vi "New_FPGA_Hex_Gen.vi"(9 "Laser(V)":dbl[](array[numeric]), 11 "Chirp Parameters":T21) -> (0 "distortion_corr":dbl, 1 "timings_offsets":dbl[](array[numeric]), 2 "HEX Array":string[](array[string]), 3 "Interrupted":bool)   [LabVIEW 2020]
uses:
  Controls/Frequency Record.ctl
  Global Variables/General Globals.vi
  Typedefs/HW config states enum.ctl
  Controls/Pockels_Galvo_Params.ctl
  Typedefs/Chirp_ABCD.ctl
  Typedefs/Cam VidRec HW config setup cluster.ctl
  Typedefs/Control Sys HW config cluster.ctl
  <vilib>/userDefined/High Color/nirio_resource_hc.ctl
  Typedefs/FPGA input type AC-DC.ctl
  Typedefs/DAQmx physical channels cluster.ctl
  Typedefs/Encoder config cluster.ctl
  Typedefs/Laser 1 config cluster.ctl
  Typedefs/PreChirper 1 config cluster.ctl
  Typedefs/Laser Power Control HW config.ctl
  Typedefs/Triggers HW config.ctl
  Typedefs/Hardware Configuration settings.ctl
  RIG-SPECIFIC FILES/FPGA Refs/FPGA Ref.ctl
  Typedefs/DAQ FPGA system config.ctl
  Typedefs/CTRL system config.ctl
  Typedefs/System Configuration.ctl
  Typedefs/DAQ FPGA HW config cluster.ctl
  Typedefs/PMT Control Voltage limits.ctl
  Peripherals Control/XYZ Stage/Control/typedefs/XYZControlConfig.ctl
  Typedefs/Comms Type.ctl
  Typedefs/Peripherals comms config cluster.ctl
panel:
  in  "System Config":T1={"Laser wavelength (nm)"=920.0, "DAQ FPGA System"={"Clock Freq (MHz) "=200.0, "Samples Wait after Trigger"=5080, "AOD fill"=4900, "StartupDelay"=0, "Slip Cycle (clock cycles)"=600000, "Add Cycle"=TRUE}, "Control system"={"AOD 1 Amplitude"=0, "AOD 2 Amplitude"=0, "AOD 3 Amplitude"=0, "AOD 4 Amplitude"=0, "AOD 5 Amplitude"=0, "AOD 6 Amplitude"=0, "T0 (ns)"=0.0, "Ta (ns)"=0.0, "Data Time Interval (ns)"=0.0, "Ctrl FPGA Clock (MHz)"=240.0}} {"Control system"."Ctrl FPGA Clock (MHz)" min=80.0 max=500.0 step=1.0; "Control system"."Data Time Interval (ns)" min=0.0 max=2048.0 step=1.0; "Control system"."Ta (ns)" min=0.0 max=2048.0 step=1.0; "Control system"."T0 (ns)" min=0.0 max=2048.0 step=1.0; "Control system"."AOD 6 Amplitude" min=0 max=2048 step=1; "Control system"."AOD 5 Amplitude" min=0 max=2048 step=1; "Control system"."AOD 4 Amplitude" min=0 max=2048 step=1; "Control system"."AOD 3 Amplitude" min=0 max=2048 step=1; "Control system"."AOD 2 Amplitude" min=0 max=2048 step=1; "Control system"."AOD 1 Amplitude" min=0 max=2048 step=1; "Laser wavelength (nm)" min=800.0 max=1080.0 step=1.0}
  in  "Hardware Config":T4={"Dev. PC"=FALSE, "Swap XY on stage"=FALSE, "No of AOD"=0, "MC Supported"=FALSE, "Axial MC"=FALSE, "Computer MAC address"="", "Externalise Triggers"=FALSE, "Trigger HW config"={"Available Device List"=0, "Device Address"=""}, "DAQmx Chan"={"Pockels AO"="", "Hard shutter AO"="", "PMT AOs"="", "Galvo AOs"="", "Power meter AI"=""}, "XYZ Stage Control Config"=enum."None", "XY stage available"=FALSE, "XY Comms Config Cluster"={"Name"="COM7", "Device Address"="", "Port "=0, "Baudrate"=0, "Comms Type"=enum."GPIB-IEEE488"}, "Y stage available"=FALSE, "Y Comms Config Cluster"={"Name"="", "Device Address"="", "Port "=0, "Baudrate"=0, "Comms Type"=enum."GPIB-IEEE488"}, "Z stage available"=FALSE, "Z Comms Config Cluster "={"Name"="", "Device Address"="", "Port "=0, "Baudrate"=0, "Comms Type"=enum."GPIB-IEEE488"}, "Encoder available"=FALSE, "Encoder"={"IP address"="224.0.1.103", "Port"=7000, "Wheel radius (cm)"=16.0, "Encoder Trigger"=""}, "VidRec available"=FALSE, "Cam VidRec"={"DO flag-Video record"="", "DO flag-Trial start"=""}, "Laser Power Control HW config"={"Laser Power Control"="", "Laser Power Modulation Control"=enum."NI"}, "Laser 1 available"=FALSE, "Laser 1 config cluster"={"COM port"="COM7", "Baud Rate"=0, "Type"=""}, "Prechirper 1 available"=FALSE, "Prechirper 1 config cluster"={"Type"="", "Baud Rate"=0, "COM port"="COM7"}, "Control system.FPGA available?"=FALSE, "Control Sys. HW config"={"Control system.FPGA Type"=enum."Virtex 5", "Control system.Network adapter name"="", "Control system.MAC address"="", "Control system.Ethernet Port"=0, "Control system.Ethernet Port Opened"=FALSE}, "DAQ FPGA HW Config"={"FGPA Ref"=refnum, "Target"="RIO0", "input card type"=enum."AC Card"}, "PMT Control Voltage Limits"={"Lower Limit"=0.0, "Upper Limit"=0.0}} {"Encoder"."Wheel radius (cm)" format="%#_13g"}
  out "difftime - aodcontrol delay":dbl
  out "diff time":dbl
  in  "frontpanel":bool
  out "Loop index":i32
  # "RE-ENTRANT"
  # "(make , model etc)"
  # "(COM Port / IP Address / service address etc.)"
  # "(Port for ethernet / channel for BT)"
  # "(make , model etc)"
  # "(COM Port / IP Address / service address etc.)"
  # "(Port for ethernet / channel for BT)"
  # "(make , model etc)"
  # "(COM Port / IP Address / service address etc.)"
  # "(Port for ethernet / channel for BT)"
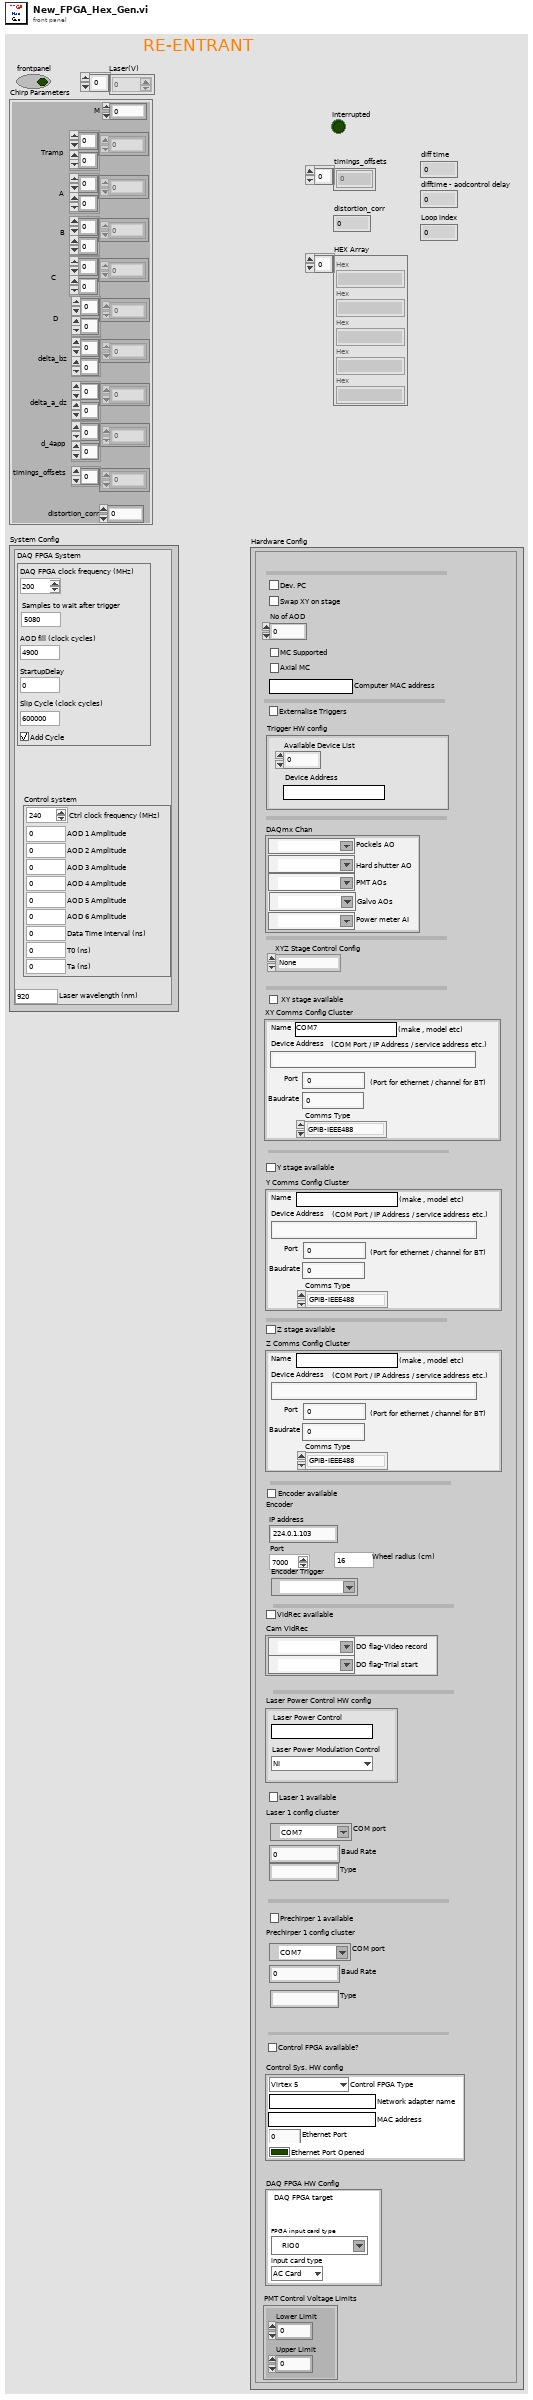
[diagram p1: front panel]
types:
  T1 = typedef "System Configuration.ctl" = cluster{"Laser wavelength (nm)":dbl, "DAQ FPGA System":T2, "Control system":T3}
  T2 = typedef "DAQ FPGA system config.ctl" = cluster{"Clock Freq (MHz) ":dbl, "Samples Wait after Trigger":u16, "AOD fill":u16, "StartupDelay":i32, "Slip Cycle (clock cycles)":u32, "Add Cycle":bool}
  T3 = typedef "CTRL system config.ctl" = cluster{"AOD 1 Amplitude":i16, "AOD 2 Amplitude":i16, "AOD 3 Amplitude":i16, "AOD 4 Amplitude":i16, "AOD 5 Amplitude":i16, "AOD 6 Amplitude":i16, "T0 (ns)":dbl, "Ta (ns)":dbl, "Data Time Interval (ns)":dbl, "Ctrl FPGA Clock (MHz)":dbl}
  T4 = typedef "Hardware Configuration settings.ctl" = cluster{"Dev. PC":bool, "Swap XY on stage":bool, "No of AOD":u8, "MC Supported":bool, "Axial MC":bool, "Computer MAC address":string, "Externalise Triggers":bool, "Trigger HW config":T5, "DAQmx Chan":T6, "XYZ Stage Control Config":T7, "XY stage available":bool, "XY Comms Config Cluster":T8, "Y stage available":bool, "Y Comms Config Cluster":T8, "Z stage available":bool, "Z Comms Config Cluster ":T8, "Encoder available":bool, "Encoder":T10, "VidRec available":bool, "Cam VidRec":T11, "Laser Power Control HW config":T12, "Laser 1 available":bool, "Laser 1 config cluster":T13, "Prechirper 1 available":bool, "Prechirper 1 config cluster":T14, "Control system.FPGA available?":bool, "Control Sys. HW config":T15, "DAQ FPGA HW Config":T16, "PMT Control Voltage Limits":T20}
  T5 = typedef "Triggers HW config.ctl" = cluster{"Available Device List":i32, "Device Address":string}
  T6 = typedef "DAQmx physical channels cluster.ctl" = cluster{"Pockels AO":tag, "Hard shutter AO":tag, "PMT AOs":tag, "Galvo AOs":tag, "Power meter AI":tag}
  T7 = typedef "XYZControlConfig.ctl" = enum16{"None", "XYZ", "XY-Z", "X-Y-Z", "Z"}
  T8 = typedef "Peripherals comms config cluster.ctl" = cluster{"Name":string, "Device Address":string, "Port ":u16, "Baudrate":i32, "Comms Type":T9}
  T9 = typedef "Comms Type.ctl" = enum16{"GPIB-IEEE488", "Serial-RS232", "Serial-RS485", "Serial-RS422", "Serial-USB", "Ethernet-TCP/IP", "Ethernet-UDP"}
  T10 = typedef "Encoder config cluster.ctl" = cluster{"IP address":string, "Port":u16, "Wheel radius (cm)":dbl, "Encoder Trigger":tag}
  T11 = typedef "Cam VidRec HW config setup cluster.ctl" = cluster{"DO flag-Video record":tag, "DO flag-Trial start":tag}
  T12 = typedef "Laser Power Control HW config.ctl" = cluster{"Laser Power Control":string, "Laser Power Modulation Control":enum16{"NI", "FPGA"}}
  T13 = typedef "Laser 1 config cluster.ctl" = cluster{"COM port":refnum<visa-resource-name>, "Baud Rate":i32, "Type":string}
  T14 = typedef "PreChirper 1 config cluster.ctl" = cluster{"Type":string, "Baud Rate":i32, "COM port":refnum<visa-resource-name>}
  T15 = typedef "Control Sys HW config cluster.ctl" = cluster{"Control system.FPGA Type":enum16{"Virtex 5", "Virtex 7"}, "Control system.Network adapter name":string, "Control system.MAC address":string, "Control system.Ethernet Port":u32, "Control system.Ethernet Port Opened":bool}
  T16 = typedef "DAQ FPGA HW config cluster.ctl" = cluster{"FGPA Ref":T17, "Target":T18, "input card type":T19}
  T17 = typedef "FPGA Ref.ctl" = refnum<k20>
  T18 = typedef "nirio_resource_hc.ctl" = tag
  T19 = typedef "FPGA input type AC-DC.ctl" = enum16{"AC Card", "DC Card"}
  T20 = typedef "PMT Control Voltage limits.ctl" = cluster{"Lower Limit":dbl, "Upper Limit":dbl}
  T21 = typedef "Chirp_ABCD.ctl" = cluster{"M ":dbl, "Tramp":dbl[][], "A":dbl[][], "B":dbl[][], "C":dbl[][], "D":dbl[][], "delta_bz":dbl[][], "delta_a_dz":dbl[][], "d_4app":dbl[][], "timings_offsets":dbl[], "distortion_corr":dbl}
  T22 = typedef "Pockels_Galvo_Params.ctl" = cluster{"A":dbl[], "Pockels Level":dbl[], "X Galvo":dbl[], "Y Galvo":dbl[], "AOD Fill Cycles":dbl[], "delta_a_dz":dbl[]}
  T23 = typedef "Frequency Record.ctl" = cluster{"Phi":dbl[], "A":dbl[], "B":dbl[], "C":dbl[], "D":dbl[], "E":dbl[], "Tstart":dbl[], "Tframe":dbl[]}
  T24 = typedef "HW config states enum.ctl" = enum16{"Load from file", "Save to file", "Save backup", "Write all", "Read all", "Write XY stage settings", "Write DAQ FPGA settings", "Write Control FPGA settings", "Write Phys Channels", "Write System Config", "Write HW Config", "Save System Config", "Save HW Config", "Clear", "Compare from file"}
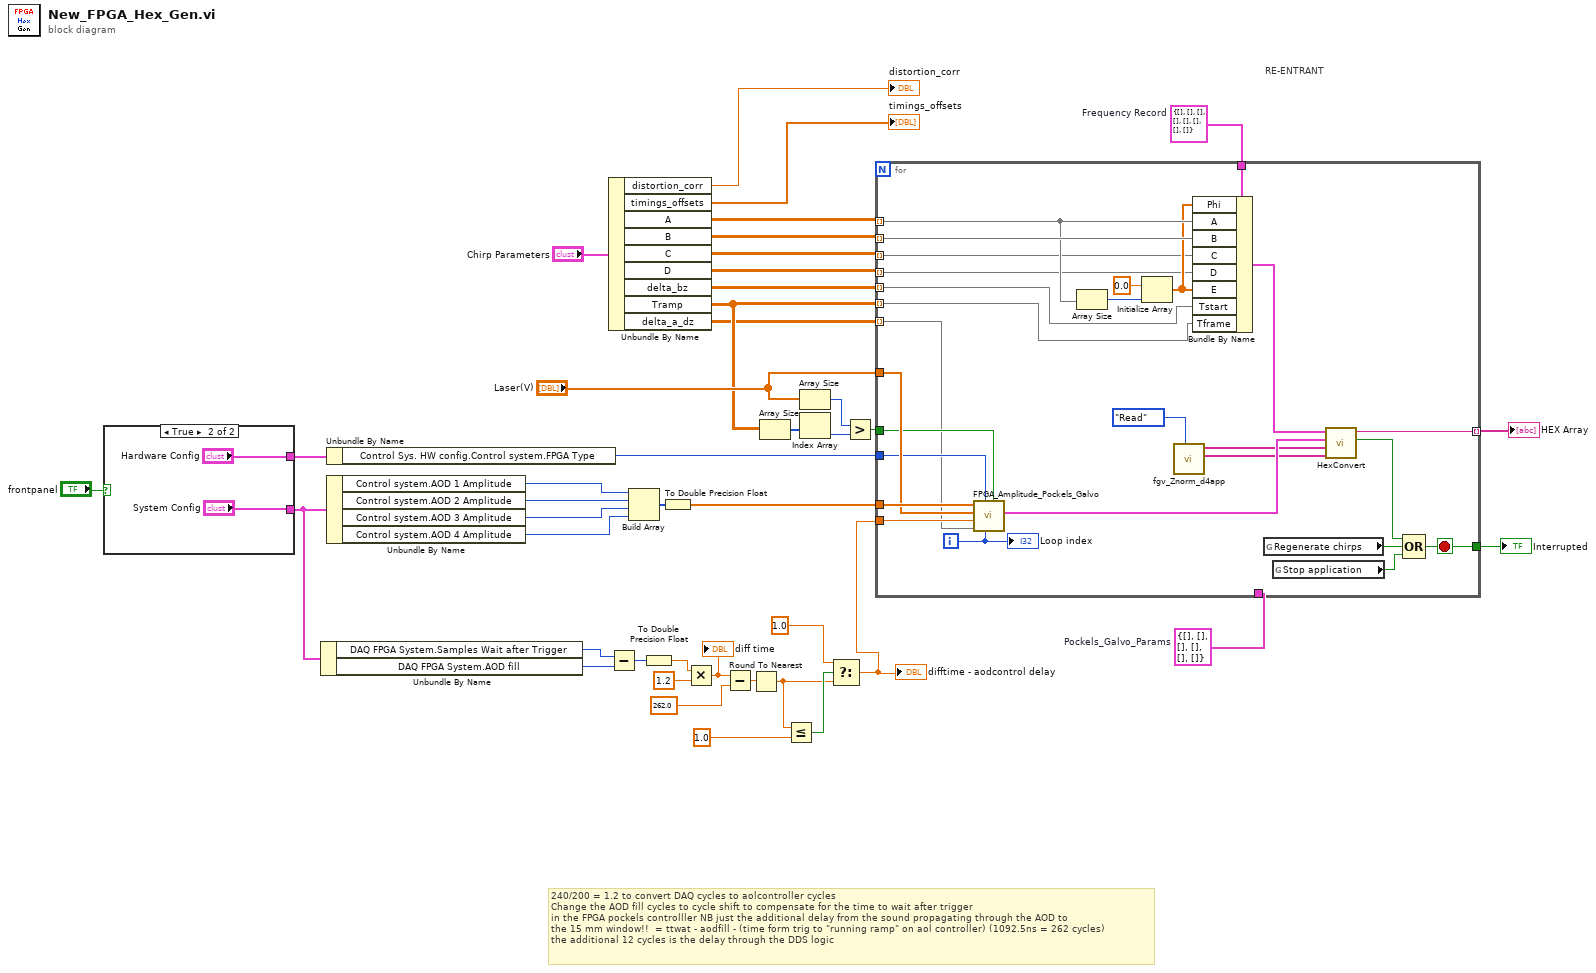
[diagram p0: block diagram]
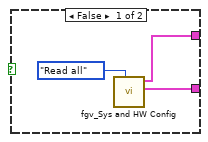
[diagram p2: hidden frame]
diagram:
  w28 = T22 {"A"=[], "Pockels Level"=[], "X Galvo"=[], "Y Galvo"=[], "AOD Fill Cycles"=[], "delta_a_dz"=[]}  # Pockels_Galvo_Params
  w42 = T23 {"Phi"=[], "A"=[], "B"=[], "C"=[], "D"=[], "E"=[], "Tstart"=[], "Tframe"=[]}  # Frequency Record
  # "240/200 = 1.2 to convert DAQ cycles to aolcontroller cycles\nChange the AOD fill cycles to cycle shift to compensate for the time to wait after trigger\nin the FPGA pockels controlller NB just the additional delay from the sound propagating through the AOD to\nthe 15 mm window!!  = ttwat - aodfill - (time form trig to \"running ramp\" on aol controller) (1092.5ns = 262 cycles)\nthe additional 12 cycles is the delay through the DDS logic"
  # "RE-ENTRANT"
  n1 = case shown="True" "frontpanel" {
    tunnel: [w44 "System Config"] -> w14
    tunnel: [w43 "Hardware Config"] -> w13
    frame False {
      n2 = call "fgv_Sys and HW Config.vi"("Function"=HW_config_states_enum."Read all") -> ("System Config OUT"=w44:T1, "Hardware Configuration OUT"=w43:T4)  [unwired: 8 in, 1 out]
    }
    frame True {
    }
  }
  n3 = Unbundle By Name(w14) -> ("DAQ FPGA System.Samples Wait after Trigger"=w23:u16, "DAQ FPGA System.AOD fill"=w22:u16)
  n4 = Unbundle By Name(w13) -> ("Control Sys. HW config.Control system.FPGA Type"=w12:enum16{"Virtex 5", "Virtex 7"})
  n5 = Unbundle By Name(w14) -> ("Control system.AOD 1 Amplitude"=w39:i16, "Control system.AOD 2 Amplitude"=w38:i16, "Control system.AOD 3 Amplitude"=w37:i16, "Control system.AOD 4 Amplitude"=w36:i16)
  n6 = Unbundle By Name("Chirp Parameters") -> ("distortion_corr"=→"distortion_corr":dbl, "timings_offsets"=→"timings_offsets":dbl[], "A"=w35:dbl[][], "B"=w11:dbl[][], "C"=w33:dbl[][], "D"=w32:dbl[][], "delta_bz"=w4:dbl[][], "Tramp"=w5:dbl[][], "delta_a_dz"=w3:dbl[][])
  n7 = Subtract(x=w23, y=w22) -> (x-y=w21:u16)
  n8 = Build Array(w39, w38, w37, w36) -> (w34:i16[])
  n9 = To Double Precision Float(number=w21) -> (double precision float=w20:dbl)
  n10 = To Double Precision Float(number=w34) -> (double precision float=w30:dbl[])
  n11 = Multiply(x=w20, y=1.2) -> (x*y=w18:dbl)
  "diff time" <- w18
  n12 = Subtract(x=w18, y=262.0) -> (x-y=w16:dbl)
  n13 = Round To Nearest(number=w16) -> (nearest integer value=w7:dbl)
  n14 = Array Size(array=w5) -> (size(s)=w27:i32[])
  n15 = Less Or Equal?(x=w7, y=1.0) -> (x <= y?=w9:bool)
  n16 = Array Size(array="Laser(V)") -> (size(s)=w25:i32)
  n17 = Index Array(array=w27) -> (element=w26:i32)  [unwired: 1 in]
  n18 = Select(t=1.0, s=w9, f=w7) -> (s? t:f=w6:dbl)
  "difftime - aodcontrol delay" <- w6
  n19 = Greater?(x=w25, y=w26) -> (0:w24:bool)
  n20 = for {
    tunnel: w35 -> [w69] mode=indexing
    tunnel: w42 -> [w71]
    tunnel: w28 -> [_]
    tunnel: w30 -> [w58]
    tunnel: w33 -> [w61] mode=indexing
    tunnel: w11 -> [w70] mode=indexing
    tunnel: w32 -> [w60] mode=indexing
    tunnel: [w67] -> w40 mode=indexing
    tunnel: [w66] -> w31
    tunnel: w5 -> [w63] mode=indexing
    tunnel: w6 -> [w56]
    tunnel: "Laser(V)" -> [w57]
    tunnel: w24 -> [w53]
    tunnel: w12 -> [w54]
    tunnel: w4 -> [w49] mode=indexing
    tunnel: w3 -> [w48] mode=indexing
    i -> [w55]
    stop <- w66 stop-if-true
    n21 = call "FPGA_Amplitude_Pockels_Galvo.vi"("Live(F)/Functional(T)"=w53, "Chirp index"=w55, "FPGA Type"=w54, "delta_a_dz"=w48, "difftime - aodcontrol delay"=w56, "Laser(V) - Vertex 7 Only"=w57, "Amplitude"=w58) -> ("Pockels_Galvo_Params"=w59:T22)  [unwired: 4 in]
    n22 = Array Size(array=w69) -> (size(s)=w72:i32)
    n23 = Initialize Array(0.0 ("element"), w72) -> (w62:dbl[])
    n24 = call "fgv_Znorm_d4app.vi"("Function"=enum16{"Idle", "Write", "Read"}."Read") -> ("E Field"=w50:string[], "Phase Field"=w51:string[])  [unwired: 8 in, 1 out]
    n25 = Bundle By Name(cluster=w71, "Phi"=w62, "A"=w69, "B"=w70, "C"=w61, "D"=w60, "E"=w62, "Tstart"=w49, "Tframe"=w63) -> (w68:T23)
    n26 = global read "General Globals.vi" "Regenerate chirps"() -> (w66:bool)
    n27 = global read "General Globals.vi" "Stop application"() -> (w64:bool)
    n28 = call "HexConvert.vi"("E Field"=w50, "Phase Field"=w51, "Pockels_Galvo_Params"=w59, "Frequency Record"=w68) -> ("Interrupted"=w65:bool, "Hex"=w67:string)  [unwired: 6 in]
    n29 = Compound Arithmetic op=OR(w65, w66, w64) -> ()  [unwired: 1 out]
    "Loop index" <- w55
  }
  "HEX Array" <- w40
  "Interrupted" <- w31
